vi "Chirp_EIS_Calculation.vi"(8 "error in (no error)":errorcluster, 11 "ChirpEIS in":refnum<class "ChirpEIS.lvclass">) -> (0 "error out":errorcluster, 1 "EIS Results":string, 2 "Show EIS Results":dbl[][](array[numeric]), 3 "ChirpEIS out":refnum<class "ChirpEIS.lvclass">)   [LabVIEW 2014, in "ChirpEIS.lvclass"]
uses:
  ChirpEIS.lvclass
  ChirpEIS.lvclass/ChirpEIS.ctl
  <vilib>/Analysis/2dsp.llb/Real FFT.vi
  <vilib>/Analysis/NI_AALPro.lvlib
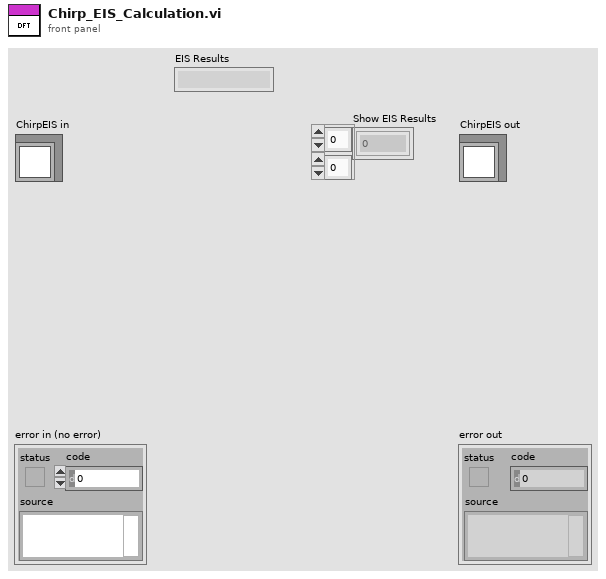
[diagram p1: front panel]
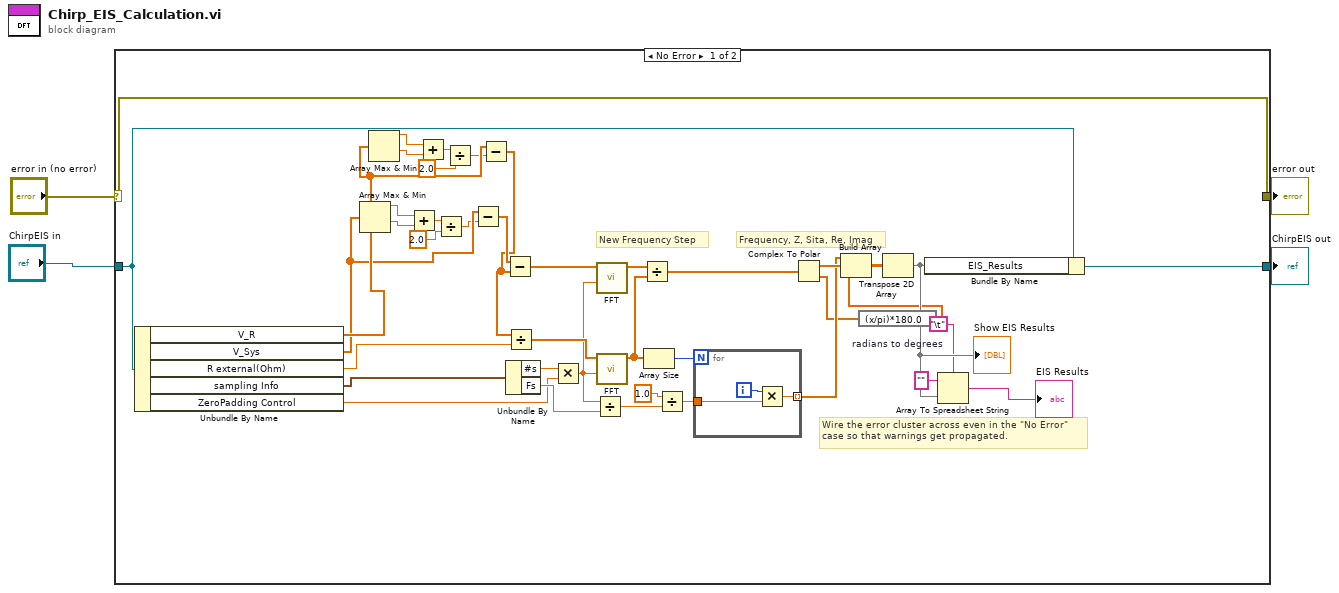
[diagram p0: block diagram]
diagram:
  n1 = case shown="No Error" "error in (no error)" {
    selector: "error in (no error)" -> [w45 w50]
    tunnel: [w45 w50] -> w3
    tunnel: [w25 w49] -> w1
    tunnel: "ChirpEIS in" -> [w26 w49]
    frame No Error {
      # "Frequency, Z, Sita, Re, Imag"
      # "New Frequency Step"
      # "Wire the error cluster across even in the \"No Error\"\ncase so that warnings get propagated."
      n2 = Unbundle By Name(w26) -> ("V_R"=w16:dbl[], "V_Sys"=w9:dbl[], "R external(Ohm)"=w27:dbl, "sampling Info"=w29:cluster{"Fs":dbl, "#s":dbl}, "ZeroPadding Control"=w28:dbl)
      n3 = Array Max & Min(array=w9) -> (max value=w7:dbl, min value=w6:dbl)  [unwired: 2 out]
      n4 = Array Max & Min(array=w16) -> (max value=w15:dbl, min value=w14:dbl)  [unwired: 2 out]
      n5 = Add(x=w7, y=w6) -> (x+y=w10:dbl)
      n6 = Add(x=w15, y=w14) -> (x+y=w13:dbl)
      n7 = Divide(x=w10, y=2.0) -> (x/y=w5:dbl)
      n8 = Divide(x=w13, y=2.0) -> (x/y=w11:dbl)
      n9 = Subtract(x=w9, y=w5) -> (x-y=w18:dbl[])
      n10 = Subtract(x=w16, y=w11) -> (x-y=w17:dbl[])
      n11 = Subtract(x=w18, y=w17) -> (x-y=w44:dbl[])
      n12 = Divide(x=w17, y=w27) -> (x/y=w40:dbl[])
      n13 = Unbundle By Name(w29) -> ("#s"=w30:dbl, "Fs"=w31:dbl)
      n14 = Multiply(x=w30, y=w28) -> (x*y=w39:dbl)
      n15 = Divide(x=w39, y=w31) -> (x/y=w32:dbl)
      n16 = call-poly <vilib>:"FFT.vi"("FFT size"=w39, "X"=w44) -> ("FFT {X}"=w41:cdb[])  [unwired: 8 in, 1 out]
      n17 = call-poly <vilib>:"FFT.vi"("FFT size"=w39, "X"=w40) -> ("FFT {X}"=w42:cdb[])  [unwired: 8 in, 1 out]
      n18 = Divide(x=w41, y=w42) -> (x/y=w43:cdb[])
      n19 = Array Size(array=w42) -> (size(s)=w35:i32)
      n20 = Divide(x=1.0, y=w32) -> (x/y=w34:dbl)
      n21 = for {
        N: w35 -> [_]
        tunnel: w34 -> [w48]
        tunnel: [w46] -> w36 mode=indexing
        i -> [w47]
        n22 = Multiply(x=w47, y=w48) -> (x*y=w46:dbl)
      }
      n23 = Complex To Polar(r * e^(i*theta)=w43) -> (r=w37:dbl[], theta=w20:dbl[])
      n24 = expression code="(x/pi)*180.0" "radians to degrees"(w20) -> (w19:dbl[])
      n25 = Build Array(w36, w37, w19) -> (w38:dbl[][])
      n26 = Transpose 2D Array(2D array=w38) -> (transposed array=w24:dbl[][])
      "Show EIS Results" <- w24
      n27 = Bundle By Name(cluster=w26, "EIS_Results"=w24) -> (w25:refnum<class "ChirpEIS.lvclass">)
      n28 = Array To Spreadsheet String(delimiter (Tab)="\t", array=w24, 3:"" ("format string")) -> (spreadsheet string=→"EIS Results":string)
    }
    frame Error {
    }
  }
  "error out" <- w3
  "ChirpEIS out" <- w1
